vi "Example Graph.vi"() -> ()   [LabVIEW 2010]
uses:
  C:/tf/play/labview/Tinkerforge.dll
panel:
  out "graph":cluster{"X":dbl, "Y":dbl}[](graph)
  in  "stop":bool
  in  "uid":string="6j9"
  in  "port":i32=4223
  in  "host":string="localhost"
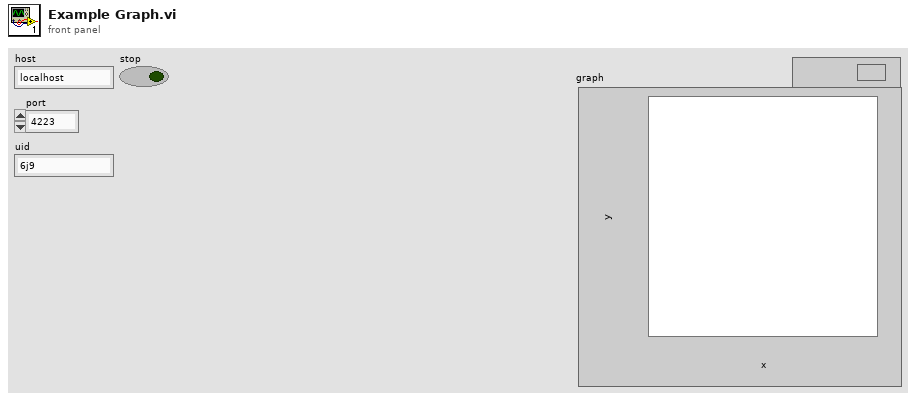
[diagram p1: front panel]
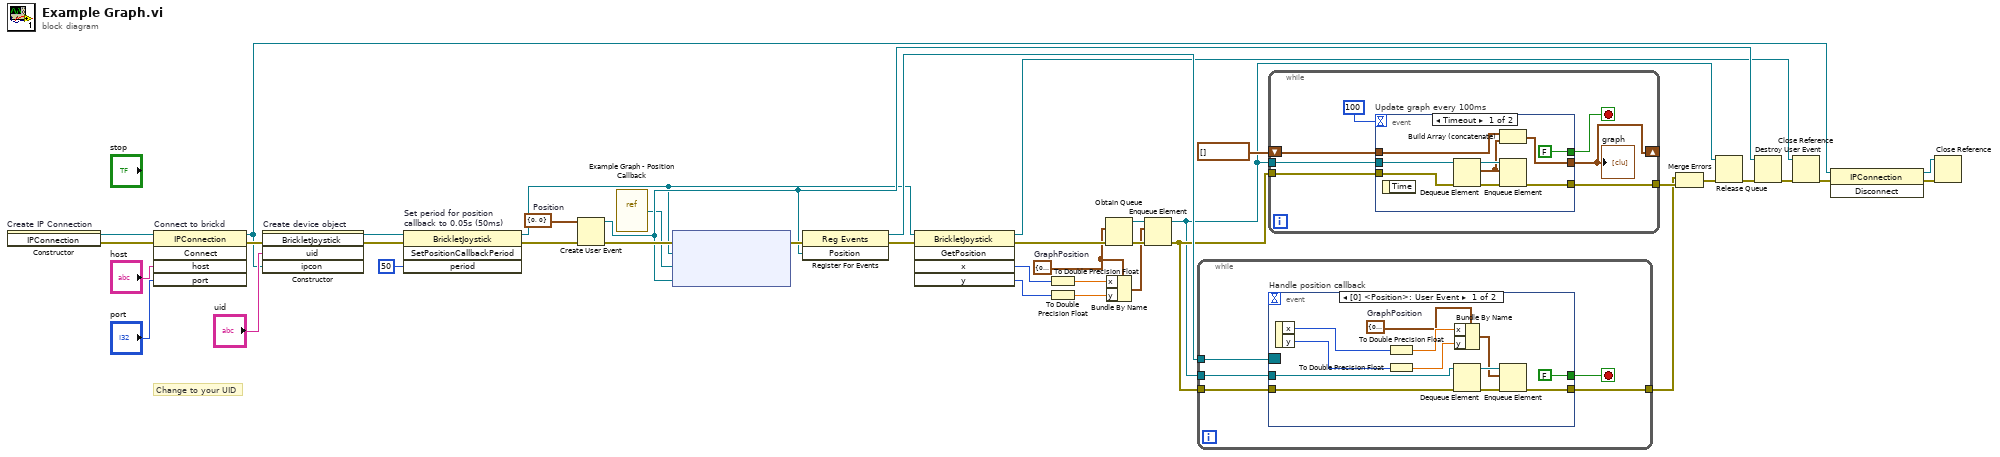
[diagram p0: block diagram]
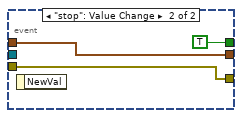
[diagram p2: hidden frame]
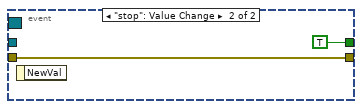
[diagram p3: hidden frame]
diagram:
  w3 = cluster{"x":dbl, "y":dbl} {"x"=0.0, "y"=0.0}  # GraphPosition
  w26 = cluster{"x":i16, "y":i16} {"x"=0, "y"=0}  # Position
  # "Change to your UID"
  n1 = constructor on="Create IP Connection" class="IPConnection"() -> (reference out=w40:refnum<k24>, error out=w12:errorcluster)  [unwired: 3 in, 1 out]
  n2 = invoke on="Connect to brickd" class="IPConnection" method="Connect"(reference=w40, error in=w12, "host"="host", "port"="port") -> (reference out=w33:refnum<k24>, error out=w36:errorcluster)  [unwired: 1 in, 3 out]
  n3 = constructor on="Create device object" class="BrickletJoystick"(error in=w36, "uid"="uid", "ipcon"=w33) -> (reference out=w23:refnum<k24>, error out=w25:errorcluster)  [unwired: 2 in, 3 out]
  n4 = invoke on="Set period for position\ncallback to 0.05s (50ms)" class="BrickletJoystick" method="SetPositionCallbackPeriod"(reference=w23, error in=w25, "period"=i64 50) -> (reference out=w9:refnum<k24>, error out=w24:errorcluster)  [unwired: 1 in, 2 out]
  n5 = Create User Event(user event datatype=w26, error in=w24) -> (user event=w28:refnum<user-event>, error out=w31:errorcluster)
  n6 = vi-ref "Example Graph - Position Callback.vi"() -> ("vi reference"=w2:refnum<vi>)
  n7 = node ("Register Event Callback")(w31, w9, w2, w28) -> (w30:errorcluster)  [unwired: 1 in, 1 out]
  n8 = register-events(error in=w30, w28) -> (reference out=w29:refnum<event-registration>, error out=w11:errorcluster)  [unwired: 1 in]
  n9 = invoke class="BrickletJoystick" method="GetPosition"(reference=w9, error in=w11) -> (reference out=w8:refnum<k24>, error out=w10:errorcluster, "x"=w5:i16, "y"=w4:i16)  [unwired: 3 in, 1 out]
  n10 = To Double Precision Float(number=w5) -> (double precision float=w7:dbl)
  n11 = To Double Precision Float(number=w4) -> (double precision float=w6:dbl)
  n12 = Obtain Queue(element data type=w3, error in (no error)=w10) -> (queue out=w16:refnum<queue>, error out=w18:errorcluster)  [unwired: 3 in, 1 out]
  n13 = Bundle By Name(cluster=w3, "x"=w7, "y"=w6) -> (w1:cluster{"x":dbl, "y":dbl})
  n14 = Enqueue Element(queue=w16, element=w1, error in (no error)=w18) -> (queue out=w13:refnum<queue>, error out=w17:errorcluster)  [unwired: 1 in, 1 out]
  n15 = while {
    tunnel: w29 -> [w45]
    tunnel: [w43] -> w20
    tunnel: w17 -> [w44]
    tunnel: w13 -> [w42]
    stop <- w41 stop-if-true
    n16 = event "Handle position callback" shown="[0] <Position>: User Event" {
      selector: w45 -> [_ _]
      dyn-events: _ -> [_ _]
      timeout: _ -> [_ _]
      tunnel: w44 -> [w57 w58]
      tunnel: [w55 w58] -> w43
      tunnel: w42 -> [w54 _]
      tunnel: [FALSE TRUE] -> w41
      event User Event {
        w46 = cluster{"x":dbl, "y":dbl} {"x"=0.0, "y"=0.0}  # GraphPosition
        n17 = event-data() -> ("x"=w49:i16, "y"=w48:i16)  [unwired: 1 in]
        n18 = To Double Precision Float(number=w49) -> (double precision float=w51:dbl)
        n19 = To Double Precision Float(number=w48) -> (double precision float=w50:dbl)
        n20 = Dequeue Element(queue=w54, error in (no error)=w57) -> (queue out=w53:refnum<queue>, error out=w56:errorcluster)  [unwired: 1 in, 2 out]
        n21 = Bundle By Name(cluster=w46, "x"=w51, "y"=w50) -> (w47:cluster{"x":dbl, "y":dbl})
        n22 = Enqueue Element(queue=w53, element=w47, error in (no error)=w56) -> (error out=w55:errorcluster)  [unwired: 1 in, 2 out]
      }
      event "stop": Value Change {
        n23 = event-data() -> ()  [unwired: 1 in, 1 out]
      }
    }
  }
  n24 = while {
    tunnel: [w63] -> w21
    tunnel: w17 -> [w64]
    shift-right: [w60] -> _
    shift-left: cluster{"x":dbl, "y":dbl}[] [] -> [w65]
    tunnel: w13 -> [w62]
    stop <- w61 stop-if-true
    n25 = event "Update graph every 100ms" shown="[0] Timeout" {
      selector: _ -> [_ _]
      dyn-events: _ -> [_ _]
      timeout: 100 -> [_ _]
      tunnel: [w75 w77] -> w60
      tunnel: w65 -> [w69 w77]
      tunnel: w64 -> [w74 w76]
      tunnel: [w71 w76] -> w63
      tunnel: w62 -> [w73 _]
      tunnel: [FALSE TRUE] -> w61
      event Timeout {
        n26 = event-data() -> ()  [unwired: 1 in, 1 out]
        n27 = Dequeue Element(queue=w73, error in (no error)=w74) -> (queue out=w70:refnum<queue>, element=w67:cluster{"x":dbl, "y":dbl}, error out=w72:errorcluster)  [unwired: 1 in, 1 out]
        n28 = Build Array (concatenate)(w69, w67) -> (w75:cluster{"x":dbl, "y":dbl}[])
        n29 = Enqueue Element(queue=w70, element=w67, error in (no error)=w72) -> (error out=w71:errorcluster)  [unwired: 1 in, 2 out]
      }
      event "stop": Value Change {
        n30 = event-data() -> ()  [unwired: 1 in, 1 out]
      }
    }
    "graph" <- w60
  }
  n31 = Merge Errors(w20, w21) -> (w15:errorcluster)
  n32 = Release Queue(queue=w13, error in (no error)=w15) -> (error out=w14:errorcluster)  [unwired: 1 in, 2 out]
  n33 = Destroy User Event(user event=w28, error in=w14) -> (error out=w27:errorcluster)
  n34 = Close Reference(reference=w8, error in (no error)=w27) -> (error out=w35:errorcluster)
  n35 = invoke class="IPConnection" method="Disconnect"(reference=w33, error in=w35) -> (reference out=w32:refnum<k24>, error out=w34:errorcluster)  [unwired: 1 in, 1 out]
  n36 = Close Reference(reference=w32, error in (no error)=w34) -> ()  [unwired: 1 out]
